vi "findNot.vi"(0 "reference in":refnum<class "Notification Controller.lvclass">, 3 "S/N:":string, 5 "error in (no error)":errorcluster) -> (14 "reference out":refnum<class "Notification Controller.lvclass">, 16 "index of element":i32, 17 "found!":bool, 19 "error out":errorcluster)   [LabVIEW 2016, in "Notification Controller.lvclass"]
uses:
  Notification Controller.lvclass
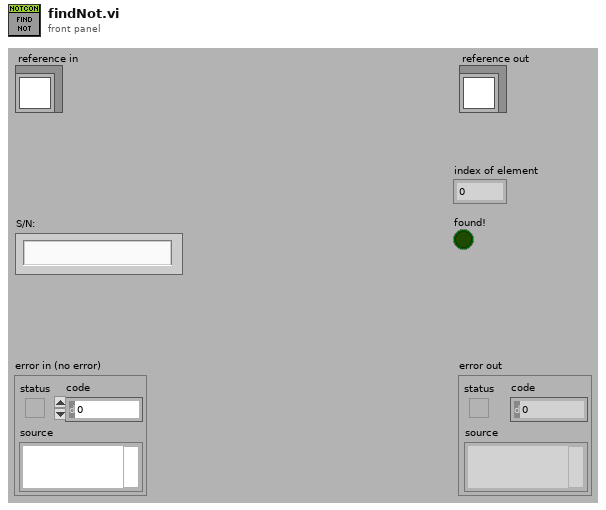
[diagram p1: front panel]
types:
  T1 = typedef "Notification Controller.lvclass/ObjectAttributesRef.ctl" = refnum<data-value>
  T2 = typedef "Notification Controller.lvclass/ObjectAttributes.ctl" = cluster{"MyAttribute":dbl, "items_data":string[][][], "items_notification_refs":refnum<class "itemsNotification.lvclass">[], "notifications_data_items":string[][], "items_nots?":bool, "devices_controller_ref":refnum<class "Devices Controller.lvclass">, "onlineUpdate":timestamp, "notController?":bool, "tracking_notification_ref":refnum<class "trackingNotification.lvclass">, "notifications_data_tracking":string[][], "tracking_parts_data":string[][], "tracking_nots?":bool, "index_tracking_not":i32[], "file_controller_ref":refnum<class "File Controller.lvclass">}
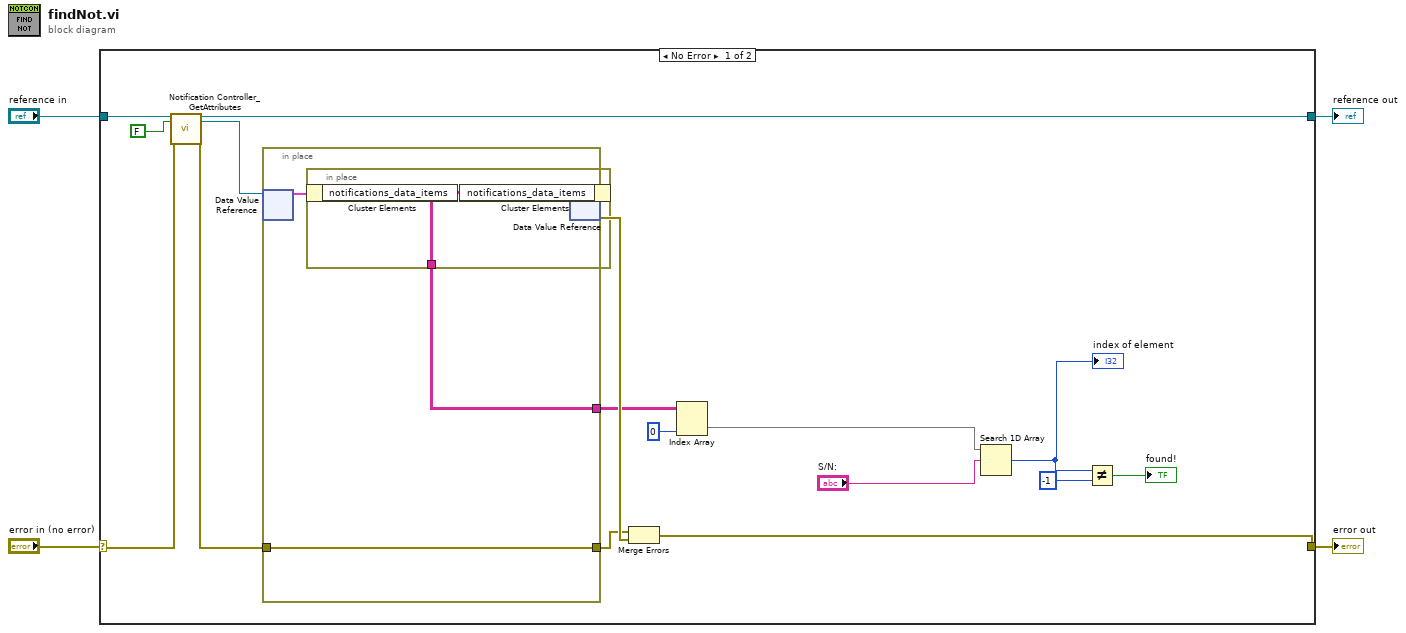
[diagram p0: block diagram]
diagram:
  n1 = case shown="No Error" "error in (no error)" {
    selector: "error in (no error)" -> [w15 w27]
    tunnel: [w20 w27] -> w3
    tunnel: [w13 w26] -> w1
    tunnel: "reference in" -> [w17 w26]
    frame No Error {
      n2 = call "Notification Controller_GetAttributes.vi"("reference in"=w17, "return data? (T)"=FALSE, "error in (no error)"=w15) -> ("reference out"=w13:refnum<class "Notification Controller.lvclass">, "attributes ref"=w12:T1, "error out"=w14:errorcluster)  [unwired: 13 in, 1 out]
      n3 = in-place {
        in-place-border: w14 -> [w22]
        in-place-border: [w22] -> w18
        in-place-border: [w21] -> w7
        n4 = in-place-dvr #1(w12) -> (w23:T2)  [unwired: 1 out]
        n5 = in-place {
          in-place-border: [w25] -> w21
          n6 = in-place-cluster #2(w23) -> ("notifications_data_items"=w25:string[][])
          n7 = in-place-cluster #2("notifications_data_items"=w25) -> (w24:T2)
        }
        n8 = in-place-dvr #1(w24) -> (w19:errorcluster)  [unwired: 1 out]
      }
      n9 = Merge Errors(w18, w19) -> (w20:errorcluster)
      n10 = Index Array(array=w7, index (col)=0 ("disabled index (col)")) -> (element=w5:string[])  [unwired: 1 in]
      n11 = Search 1D Array(1D array=w5, element="S/N:") -> (index of element=w10:i32)  [unwired: 1 in]
      "index of element" <- w10
      n12 = Not Equal?(x=w10, y=-1) -> (x != y?=→"found!":bool)
    }
    frame Error {
    }
  }
  "error out" <- w3
  "reference out" <- w1
